vi "Write Directory.vi"(8 "error in (no error)":errorcluster, 10 "Directory":path, 11 "Process Generator in":refnum<class "Process Generator.lvclass">) -> (0 "error out":errorcluster, 3 "Process Generator out":refnum<class "Process Generator.lvclass">)   [LabVIEW 2020, in "Process Generator.lvclass"]
uses:
  Process Generator.lvclass
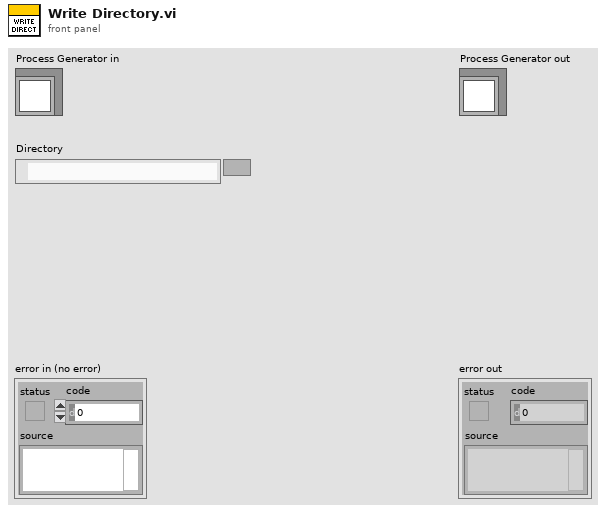
[diagram p1: front panel]
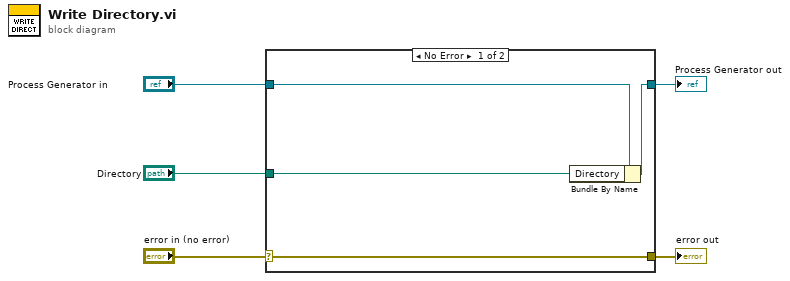
[diagram p0: block diagram]
diagram:
  n1 = case shown="No Error" "error in (no error)" {
    selector: "error in (no error)" -> [w9 w10]
    tunnel: [w9 w10] -> w4
    tunnel: [w7 w11] -> w2
    tunnel: "Process Generator in" -> [w8 w11]
    tunnel: "Directory" -> [w6 _]
    frame No Error {
      n2 = Bundle By Name(cluster=w8, "Directory"=w6) -> (w7:refnum<class "Process Generator.lvclass">)
    }
    frame Error {
    }
  }
  "error out" <- w4
  "Process Generator out" <- w2
